vi "TEST Control Value To Registry.vi"() -> ()   [LabVIEW 2013, in "Carya Config.lvclass"]
doc: "Copyright 2018, Carya Automatisering, Wiebe Walstra."
uses:
  Carya Config.lvclass
  CConfig Ctrl Ref Accessor/Registry Ctrl Ref Accessor.lvclass
  Carya Config (By Reference)/Carya Config (By Reference).lvclass
  Carya Config (By Reference)/CConfig Buffer Type/CConfig By Ref Buffer/CConfig By Ref Buffer.lvclass
panel:
  in  "Paths_Initial Scan File Path":path
  out "data":T1
  out "error out":errorcluster
  out "String":string
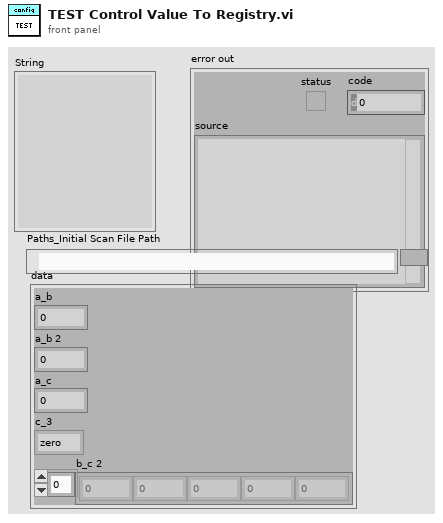
[diagram p1: front panel]
types:
  T1 = cluster{"a_b":i32, "a_b 2":i32, "a_c":csg, "c_3":enum16{"zero", "one", "two"}, "b_c 2":sgl[]}
  T2 = cluster{"a_b":i32, "a_b 2":i32, "a_c":csg, "c_3":enum16{"zero", "one", "two"}, "b_c 2":sgl[], "Paths_Initial Scan File Path":path}
  T3 = cluster{"a_q":i32[], cluster{"a_b":i32, "a_b 2":i32, "a_c":csg, "c_3":enum16{"zero", "one", "two"}, "b_c 2":sgl[], "Paths_Initial Scan File Path":path}}
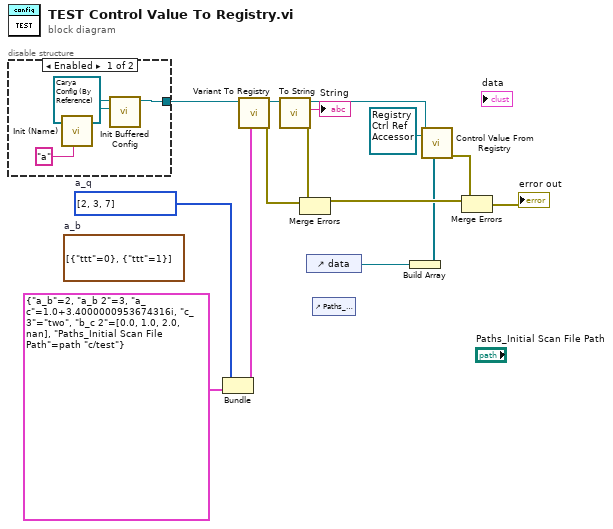
[diagram p0: block diagram]
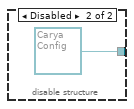
[diagram p2: hidden frame]
diagram:
  (unwired) cluster{"ttt":i32}[] [{"ttt"=0}, {"ttt"=1}]  # a_b
  w7 = i32[] [2, 3, 7]  # a_q
  n1 = disable-structure shown="Enabled" {
    disable-tunnel: [w16 refnum<class "Carya Config.lvclass"> refnum ("Carya Config in")] -> w1
    frame Enabled {
      n2 = call "Init (Name).vi"("Name"="a") -> ("Carya Config (Buffer) out"=w18:refnum<class "CConfig By Ref Buffer.lvclass">)  [unwired: 8 in, 2 out]
      n3 = call-dynamic "Init Buffered Config.vi"("Buffer Type"=w18, "Carya Config in"=refnum<class "Carya Config (By Reference).lvclass"> refnum) -> ("Carya Config out"=w16:refnum<class "Carya Config (By Reference).lvclass">)  [unwired: 8 in, 1 out]
    }
    frame Disabled {
    }
  }
  n4 = Bundle("a_q"=w7, T2 {"a_b"=2, "a_b 2"=3, "a_c"=1.0+3.4i, "c_3"=enum."two", "b_c 2"=[0.0, 1.0, 2.0, nan], "Paths_Initial Scan File Path"=path "c:/test"}) -> (w9:T3)  [unwired: 1 in]
  n5 = call "Variant To Registry.vi"("Variant"=w9, "Carya Config in"=w1) -> ("error out"=w12:errorcluster, "Carya Config out"=w15:refnum<class "Carya Config (By Reference).lvclass">)  [unwired: 6 in, 2 out]
  n6 = call-dynamic "To String.vi"("Carya Config in"=w15) -> ("error out"=w13:errorcluster, "String"=→"String":string, "Carya Config out"=w5:refnum<class "Carya Config (By Reference).lvclass">)  [unwired: 8 in]
  n7 = Merge Errors(w12, w13) -> (w11:errorcluster)
  n8 = control-ref of="data"() -> (w2:refnum<vi>)
  n9 = control-ref of="Paths_Initial Scan File Path"() -> ()  [unwired: 1 out]
  n10 = Build Array(w2) -> (w4:refnum<vi>[])
  n11 = call "Control Value From Registry.vi"("Controls"=w4, "Registry Control Reference Accessor (optional)"=refnum<class "Registry Ctrl Ref Accessor.lvclass"> refnum ("Registry Control Reference Accessor.lvclass"), "Registry Object in"=w5) -> ("error out"=w3:errorcluster)  [unwired: 6 in, 2 out]
  n12 = Merge Errors(w11, w3) -> (→"error out":errorcluster)
